vi "get_time_stamp.vi"(8 "error in (no error)":errorcluster, 11 "MeasurementResult in":refnum<class "MeasurementDatalvclass.lvclass">) -> (0 "error out":errorcluster, 2 "time_stamp":timestamp, 3 "MeasurementResult out":refnum<class "MeasurementDatalvclass.lvclass">)   [LabVIEW 2017, in "MeasurementDatalvclass.lvclass"]
doc: "Get the time stamp of measurement"
uses:
  MeasurementDatalvclass.lvclass
  MeasurementDatalvclass.lvclass/MeasurementDatalvclass.ctl
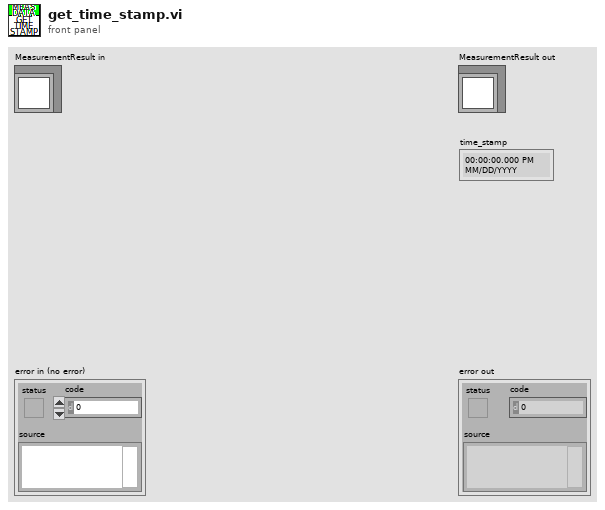
[diagram p1: front panel]
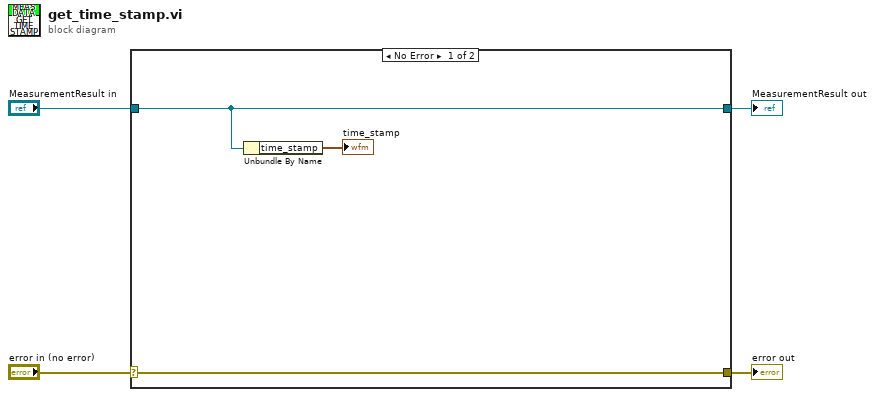
[diagram p0: block diagram]
diagram:
  n1 = case shown="No Error" "error in (no error)" {
    selector: "error in (no error)" -> [w7 w9]
    tunnel: [w7 w9] -> w3
    tunnel: [w6 w8] -> w1
    tunnel: "MeasurementResult in" -> [w6 w8]
    frame No Error {
      n2 = Unbundle By Name(w6) -> ("time_stamp"=→"time_stamp":timestamp)
    }
    frame Error {
    }
  }
  "error out" <- w3
  "MeasurementResult out" <- w1
